vi "Execute-sequences.vi"(8 "error in (no error)":errorcluster, 9 "Activity log":refnum<user-event>, 10 "Abort":refnum<notifier>, 11 "Available motors in":refnum<class "Motor-assembly.lvclass">) -> (0 "error out":errorcluster, 3 "Available motors out":refnum<class "Motor-assembly.lvclass">)   [LabVIEW 2013, in "PowderDeposition.lvlib" / "Motor-assembly.lvclass"]
uses:
  Motor-assembly.lvclass
  Motor-assembly.lvclass/Motor-assembly.ctl
  Motor/Motor.lvclass
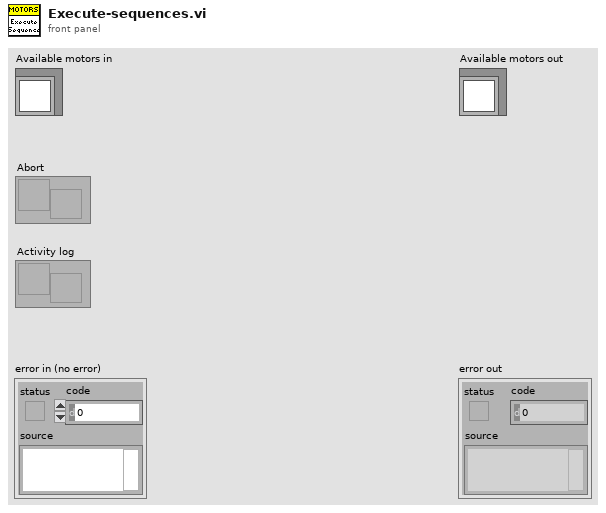
[diagram p1: front panel]
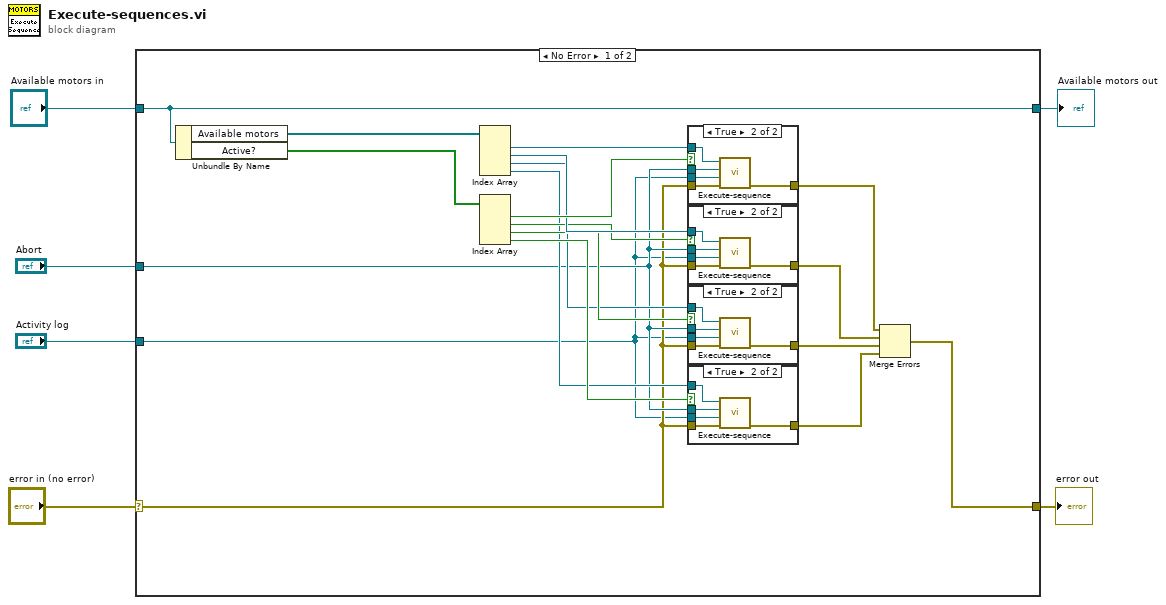
[diagram p0: block diagram]
diagram:
  n1 = case shown="No Error" "error in (no error)" {
    selector: "error in (no error)" -> [w9 w51]
    tunnel: [w8 w51] -> w5
    tunnel: [w25 w50] -> w3
    tunnel: "Available motors in" -> [w25 w50]
    tunnel: "Abort" -> [w10 _]
    tunnel: "Activity log" -> [w7 _]
    frame No Error {
      n2 = Unbundle By Name(w25) -> ("Available motors"=w24:refnum<class "Motor.lvclass">[], "Active?"=w23:bool[])
      n3 = Index Array(array=w24) -> (element #1=w22:refnum<class "Motor.lvclass">, element #2=w20:refnum<class "Motor.lvclass">, element #3=w16:refnum<class "Motor.lvclass">, element #4=w15:refnum<class "Motor.lvclass">)  [unwired: 4 in]
      n4 = Index Array(array=w23) -> (element #1=w21:bool, element #2=w19:bool, element #3=w18:bool, element #4=w17:bool)  [unwired: 4 in]
      n5 = case shown="True" w21 {
        tunnel: w22 -> [_ w49]
        tunnel: [w44 w48] -> w14
        tunnel: w10 -> [_ w47]
        tunnel: w9 -> [w44 w46]
        tunnel: w7 -> [_ w45]
        frame False {
        }
        frame True {
          n6 = call-dynamic "Execute-sequence.vi"("error in (no error)"=w46, "Activity log"=w45, "Abort"=w47, "Motor in"=w49) -> ("error out"=w48:errorcluster)  [unwired: 6 in, 1 out]
        }
      }
      n7 = case shown="True" w19 {
        tunnel: w20 -> [_ w43]
        tunnel: [w38 w42] -> w13
        tunnel: w10 -> [_ w41]
        tunnel: w9 -> [w38 w40]
        tunnel: w7 -> [_ w39]
        frame False {
        }
        frame True {
          n8 = call-dynamic "Execute-sequence.vi"("error in (no error)"=w40, "Activity log"=w39, "Abort"=w41, "Motor in"=w43) -> ("error out"=w42:errorcluster)  [unwired: 6 in, 1 out]
        }
      }
      n9 = case shown="True" w18 {
        tunnel: w16 -> [_ w31]
        tunnel: [w26 w30] -> w12
        tunnel: w10 -> [_ w29]
        tunnel: w9 -> [w26 w28]
        tunnel: w7 -> [_ w27]
        frame False {
        }
        frame True {
          n10 = call-dynamic "Execute-sequence.vi"("error in (no error)"=w28, "Activity log"=w27, "Abort"=w29, "Motor in"=w31) -> ("error out"=w30:errorcluster)  [unwired: 6 in, 1 out]
        }
      }
      n11 = case shown="True" w17 {
        tunnel: w15 -> [_ w37]
        tunnel: [w32 w36] -> w11
        tunnel: w10 -> [_ w35]
        tunnel: w9 -> [w32 w34]
        tunnel: w7 -> [_ w33]
        frame False {
        }
        frame True {
          n12 = call-dynamic "Execute-sequence.vi"("error in (no error)"=w34, "Activity log"=w33, "Abort"=w35, "Motor in"=w37) -> ("error out"=w36:errorcluster)  [unwired: 6 in, 1 out]
        }
      }
      n13 = Merge Errors(w14, w13, w12, w11) -> (w8:errorcluster)
    }
    frame Error {
    }
  }
  "error out" <- w5
  "Available motors out" <- w3
